vi "DataBuffer.vi"(0 "File Info In":T1={"FilePath"=path "/opticsmac/Users/Data", "Field (T)"=0.0, "Temperature (K)"=-1.0, "X-Axis"=enum."nm", "Center nm"=500.0, "Current Grating Density"=enum."600", "CCD Parameters"={"Exposure Time (s)"=0.2, "Offset"=0.0, "BkgrdCrct"=FALSE, "Shutter"=FALSE, "Mode"=enum."Regular", "Repetition"=4, "dt or s"=0.0}, "Operation Mode"=enum."NML Data Acquisition", "Exp Index"=0, "Index_repetition"=0, "Index"=0, "Current Detector"=enum."CCD-1024x256"} {"CCD Parameters"."dt or s" format="%#.6f"; "CCD Parameters"."Repetition" min=1; "CCD Parameters"."Offset" format="%#.2f"; "CCD Parameters"."Exposure Time (s)" min=0.02 max=6000.0 format="%#.2f"; "Center nm" format="%.2f"; "Temperature (K)" format="%.2f"; "Field (T)" format="%.2f"}, 1 "Plot Buffer Size":i32=10, 2 "Action":T7(ring) caption="Pass(0)/Write(1)/Read(2)/Init(3)", 3 "Read#":i32=1, 5 "Y Array In":dbl[](array[numeric])=[4.359859227115864, 4.389200892828675, 4.418863708420512, 4.448852482615925, 4.479172114380057, 4.509827594937488, 4.540824009842933, 4.572166541105726, 4.6038604693694944, 4.635911176148454, 4.668324146122441, 4.701104969491852, 4.734259344394734, 4.767793079387671, 4.801712095992179, 4.83602243130902, 4.870730240701915, 4.905841800553186, 4.941363511093324, 4.97730189930649, 5.0136636219147634, 5.050455468442887, 5.087684364366512, 5.125357374346244, 5.16348170554992, 5.202064711066347, 5.241113893412698, 5.280636908138933, 5.320641567532123, 5.361135844423454, 5.40212787610175, 5.443625968336108, 5.485638599511655, 5.528174424881744, 5.571242280940019, 5.614851189916724, 5.659010364402478, 5.703729212104152, 5.749017340736845, 5.79488456305601, 5.8413409020348865, 5.888396596191121, 5.936062105068024, 5.984348114875219, 6.033265544293544, 6.082825550450229, 6.133039535069095, 6.1839191508021365, 6.235476307748183, 6.287723180164464, 6.340672213378188, 6.394336130903802, 6.44872794177352, 6.5038609480878895, 6.55974875279337, 6.616405267695311, 6.673844721713221, 6.732081669387259, 6.79113099964405, 6.851007944830221, 6.9117280900235425, 6.9733073826300265, 7.0357621422775445, 7.099109071015688, 7.1633652638319365, 7.228548219495836, 7.294675851741292, 7.36176650079951, 7.429838945294219, 7.498912414511272, 7.569006601056504, 7.640141673914049, 7.7123382919199805, 7.785617617665268, 7.860001331842512, 7.935511648052952, 8.012171328088485, 8.090003697706326, 8.169032662913095, 8.249282726775652, 8.33077900677827, 8.413547252743905, 8.49761386534048, 8.58300591519227, 8.66975116261715, 8.757878078012872, 8.847415862913794, 8.93839447174277, 9.030844634282277, 9.124797878889435, 9.220286556482478, 9.317343865324164, 9.41600387663149, 9.516301561040184, 9.618272815953393, 9.721954493806981, 9.827384431281825, 9.934601479497585, 10.043645535221685, 10.154557573128157, 10.267379679144385, 10.382155084921548, 10.498928203469083, 10.617744665992642, 10.738651359976075, 10.861696468551548, 10.986929511199559, 11.114401385825383, 11.244164412257609, 11.376272377215363, 11.510780580794803, 11.647745884522498, 11.787226761028752, 11.929283345392315, 12.073977488209161, 12.22137281044176, 12.371534760102007, 12.524530670826199, 12.680429822398747, 12.83930350328164, 13.001225075210728, 13.166270039915263, 13.33451610802253, 13.506043270206384, 13.680933870638214, 13.859272682802093, 14.041146987729777, 14.226646654715656, 14.41586422456719, 14.608894995444231, 14.80583711134241, 15.00679165326711, 15.211862733147012, 15.421157590528683, 15.634786692088575, 15.852863833997525, 16.075506247159804, 16.302834705347756, 16.534973636240313, 16.77205123536335, 17.014199582923293, 17.261554763504943, 17.51425698859712, 17.77245072188844, 18.036284807256397, 18.3059125993568, 18.58149209668873, 18.863186076991337, 19.15116223479378, 19.445593320905605, 19.746657283603096, 20.054537411216362, 20.369422475784297, 20.691506877387, 21.02099078870748, 21.35808029931693, 21.702987559097092, 22.0559309201451, 22.417135076413132, 22.786831200239348, 23.165257074828247, 23.552657221611106, 23.949283021300772, 24.35539282730692, 24.771252070023422, 25.197133350337953, 25.63331652051566, 26.080088750418582, 26.537744576792313, 27.006585933108887, 27.486922157200187, 27.979069973614642, 28.48335344733274, 29.000103905129734, 29.52965982050742, 30.072366657732513, 30.628576670076946, 31.198648646914766, 31.78294760382926, 32.38184440935961, 32.99571534146977, 33.624941566211746, 34.26990853044752, 34.931005259824005, 35.60862355250491, 36.3031570584605, 37.01500023335454, 37.74454715533088, 38.49219019221989, 39.25831850591429, 40.04331637991872, 40.847561355318334, 41.67142215974196, 42.51525641324812, 43.37940809451772, 44.26420475032537, 45.169954430957425, 46.09694233418251, 47.04542714051036, 48.015637022906574, 49.00776531492666, 50.02196582239054, 51.05834776541544, 52.11697033983435, 53.19783688989854, 54.30088868779076, 55.42599831987955, 56.57296268504168, 57.74149561674433, 58.931220148080584, 60.1416604476788, 61.37223346434939, 62.622240329675115, 63.890857580390986, 65.17712827640742, 66.4799531056599, 67.79808158341963, 69.1301034712415, 70.47444055896403, 71.82933897185566, 73.19286218368788, 74.56288493456158, 75.93708826921247, 77.31295592634606, 78.68777232151824, 80.05862237420615, 81.42239343285824, 82.77577954893358, 84.11528834098996, 85.43725067181454, 86.73783333448564, 88.0130549062849, 89.25880488223545, 90.4708661424704, 91.64494074005955, 92.77667891917588, 93.86171118887495, 94.89568318741601, 95.87429297840674, 96.79333032630886, 97.64871740856572, 98.43655033863818, 99.15314080272404, 99.79505705677101, 100.35916349333694, 100.84265797303367, 101.24310612502882, 101.55847185679316, 101.78714337508754, 101.92795410705088, 101.98019801980197, 101.94363896561752, 101.81851382289437, 101.60552935527126, 101.30585286653462, 100.92109688110092, 100.4532982230126, 99.90489199503531, 99.27868106899476, 98.57780178535918, 97.80568662187997, 96.96602462681605, 96.06272042200558, 95.09985256623146, 94.08163203227065, 93.01236149485176, 91.89639605523514, 90.73810594515385, 89.54184166257876, 88.31190189802533, 87.05250451647399, 85.76776076963034, 84.461652828644, 83.13801465065819, 81.8005161249856, 80.4526503871352, 79.09772414177037, 77.73885079871027, 76.37894619898024, 75.02072668985214, 73.66670929786417, 72.31921374603169, 70.98036606460397, 69.65210355285129, 68.33618086133153, 67.03417697891065, 65.74750292571056, 64.47740997120414, 63.22499821536264, 61.99122538944135, 60.77691575122682, 59.582768967111335, 58.40936888981143, 57.25719215587677, 56.12661654114332, 55.017929024924804, 53.93133352507879, 52.86695827602707, 51.82486283053664, 50.80504467356964, 49.807445442875476, 48.831956756394504, 47.87842565094678, 46.94665964030745, 46.036431403641515, 45.14748311748012, 44.27953044611727, 43.43226620646358, 42.6053637241895, 41.79847989842212, 41.011257992390064, 40.243330167348105, 39.49431977680977, 38.763843437704175, 38.05151289452863, 37.356936691921696, 36.67972167041139, 36.01947429933415, 35.37580186017517, 34.74831349280977, 34.13662111634363, 33.540340235512275, 32.959090642839186, 32.39249702604861, 31.840189489538492, 31.301803998049735, 30.7769827500592, 30.265374487814174, 29.76663475037882, 29.28042607553899, 28.80641815591104, 28.344287954158954, 27.893719781782664, 27.454405345555568, 27.026043765322786, 26.608341566525006, 26.201012650514798, 25.803778245431467, 25.41636684014538, 25.03851410354023, 24.669962791171823, 24.31046264115136, 23.95977026090333, 23.61764900628636, 23.28386885441087, 22.95820627133951, 22.640444075739502, 22.330371299429107, 22.027783045661604, 21.73248034589445, 21.444270015698585, 21.16296451039404, 20.888381780917932, 20.620345130372943, 20.35868307164673, 20.10322918643533, 19.853821985965663, 19.61030477366188, 19.372525509968213, 19.140336679507016, 18.913595160715975, 18.692162098089153, 18.475902777115053, 18.26468650198858, 18.058386476154528, 17.856879685719345, 17.660046785759945, 17.467771989538537, 17.279942960625498, 17.09645070792191, 16.917189483561163, 16.742056683667286, 16.570952751935298, 16.403781085997196, 16.240447946532107, 16.080862369071976, 15.924936078455998, 15.772583405879114, 15.623721208481035, 15.478268791420303, 15.336147832373733, 15.197282308405232, 15.061598425142755, 14.929024548204785, 14.799491136817574, 14.672930679561734, 14.549277632191464, 14.428468357465825, 14.310441066935024, 14.195135764625045, 14.08249419256267, 13.972459778087526, 13.864977582895126, 13.759994253758327, 13.657457974875705, 13.557318421794335, 13.459526716859063, 13.364035386138228, 13.27079831777925, 13.179770721748449, 13.090909090909092, 13.004171163395661, 12.91951588624077, 12.836903380214224, 12.75629490583483, 12.677652830515154, 12.600940596803213, 12.526122691683634, 12.453164616903683, 12.38203286029049, 12.312694868025606, 12.24511901784625, 12.179274593141457, 12.115131757913815, 12.05266153257834, 11.99183577056985, 11.932627135733041, 11.87500908046845, 11.818955824609674, 11.76444233500797, 11.711444305800104, 11.65993813933795, 11.60990092775727, 11.561310435165108, 11.514145080425847, 11.468383920525726, 11.424006634497912, 11.380993507889265, 11.339325417751663, 11.298983818141277, 11.259950726108972, 11.222208708166901, 11.185740867215678, 11.150530829917827, 11.116562734503766, 11.083821218996304, 11.052291409841342, 11.021958910931758, 10.992809793012693, 10.964830583456795, 10.938008256397914, 10.912330223212965, 10.887784323341283, 10.864358815431716, 10.842042368808027, 10.820824055243078, 10.800693341033405, 10.781640079365355, 10.763654502964759, 10.746727217022421, 10.730849192387653, 10.716011759022894, 10.702206599712252, 10.689425744017434, 10.677661562474725, 10.666906761026693, 10.657154375683012, 10.648397767404552, 10.640630617205472, 10.633846921468175, 10.628040987466086, 10.623207429089685, 10.619341162771164, 10.616437403603506, 10.61449166164985, 10.613499738439238, 10.613457723645045, 10.614361991942566, 10.616209200042398, 10.61899628389644, 10.622720456073516, 10.627379203301786, 10.632970284175236, 10.639491727021781, 10.646941827930538, 10.65531914893617, 10.664622516358094, 10.674851019292753, 10.68600400825716, 10.698081093981964, 10.711082146352725, 10.725007293497864, 10.73985692102218, 10.755631671384794, 10.77233244342051, 10.789960392003877, 10.808516927855083, 10.828003717487244, 10.848422683294594, 10.869776003781105, 10.892066113929618, 10.91529570571105, 10.939467728734005, 10.96458539103486, 10.990652160008423, 11.01767176347996, 11.045648190918651, 11.074585694793534, 11.104488792072516, 11.135362265865236, 11.167211167211168, 11.20004081701363, 11.233856808121402, 11.268665007559191, 11.304471558908258, 11.341282884839375, 11.379105689799312, 11.41794696285327, 11.457813980685149, 11.498714310757618, 11.540655814634878, 11.583646651469962, 11.62769528165972, 11.672810470670129, 11.719001293034513, 11.766277136528466, 11.814647706523917, 11.864123030526423, 11.914713462898968, 11.966429689775758, 12.019282734170648, 12.073283961283387, 12.12844508400873, 12.184778168652574, 12.242295640859474, 12.301010291757152, 12.360935284322133, 12.42208415997257, 12.48447084539341, 12.548109659599271, 12.613015321241827, 12.679202956166797, 12.746688105227863, 12.815486732363786, 12.885615232945288, 12.957090442399794, 13.029929645120367, 13.104150583667508, 13.179771468271484, 13.256810986643078, 13.335288314102453, 13.415223124033782, 13.496635598676047, 13.579546440259186, 13.66397688249509, 13.749948702434974, 13.837484232702424, 13.926606374114439, 14.017338608701486, 14.109705013137976, 14.203730272596845, 14.299439695039455, 14.396859225955392, 14.4960154635654, 14.596935674501095, 14.699647809977643, 14.804180522472912, 14.910563182930376, 15.018825898501593, 15.128999530844538, 15.241115714996932, 15.355206878840859, 15.471306263179047, 15.589447942441705, 15.709666846043369, 15.831998780412336, 15.956480451712276, 16.08314948928004, 16.212044469802226, 16.343204942253628, 16.47667145362424, 16.612485575458262, 16.750689931233456, 16.89132822460762, 17.034445268559747, 17.180087015457268, 17.328300588077308, 17.479134311615432, 17.632637746713556, 17.78886172353971, 17.9478583769566, 18.109681182812103, 18.274384995391078, 18.442026086065923, 18.612662183184362, 18.786352513237837, 18.963157843349737, 19.143140525129375, 19.326364539935806, 19.51289554559672, 19.70280092463277, 19.896149834033558, 20.09301325663871, 20.29346405417522, 20.49757702200397, 20.705428945633606, 20.917098659055448, 21.13266710496104, 21.35221739690145, 21.57583488344913, 21.803607214428858, 22.03562440927946, 22.27197892761611, 22.51276574206055, 22.758082413407966, 23.008029168205347, 23.262708978810554, 23.522227646009927, 23.786693884269244, 24.056219409693583, 24.3309190307785, 24.610910742027375, 24.896315820519412, 25.187258925508026, 25.483868201129862, 25.786275382310958, 26.09461590394749, 26.409029013447665, 26.729657886715053, 27.05664974765271, 27.39015599127249, 27.73033231048255, 28.077338826633632, 28.431340223896083, 28.79250588753546, 29.161010046158022, 29.537031917981217, 29.920755861189793, 30.31237152842447, 30.71207402544193, 31.120064073983663, 31.536548178868856, 31.961738799326668, 32.395854524562374, 32.83912025353589, 33.291767378922756, 33.75403397519474, 34.22616499074848, 34.70841244397801, 35.20103562315853, 35.70430128998762, 36.21848388658109, 36.743865745697, 37.2807373039094, 37.82939731740552, 38.39015308003834, 38.96332064319138, 39.54922503696516, 40.14820049211286, 40.76059066207344, 41.386748844375965, 42.0270382005743, 42.681831973785435, 43.35151370277646, 44.03647743141852, 44.73712791219888, 45.453880802309456, 46.18716285068311, 46.937412074152704, 47.705077920707076, 48.49062141761412, 49.29451530191956, 50.11724413059322, 50.95930436729756, 51.821204442444625, 52.70346478289072, 53.60661780723075, 54.53120788228832, 55.47779123595873, 56.44693582110416, 57.43922112472759, 58.45523791609419, 59.495587926931485, 60.56088345621398, 61.651746891388925, 62.76881013723119, 63.91271394274945, 65.08410711582407, 66.28364561441893, 67.51199150234996, 68.76981175672066, 70.05777691316518, 71.37655953411455, 72.72683248428955, 74.1092669966185, 75.52453051079203, 76.97328426561938, 78.45618062540582, 79.97386011959668, 81.52694817404465, 83.11605151148629, 84.7417541980828, 86.4046133123965, 88.10515421280739, 89.84386537927608, 91.62119280559367, 93.43753391876069, 95.29323100317171, 97.1885641087292, 99.12374342407416, 101.0989010989011, 103.11408250278154, 105.16923691237619, 107.26420762426427, 109.39872149710654, 111.5723779346085, 113.78463732972462, 116.03480900108816, 118.32203866462099, 120.64529549690151, 123.0033588622068, 125.39480479205825, 127.81799232482636, 130.27104983316252, 132.75186148874656, 135.25805403686783, 137.78698407721993, 140.33572607186628, 142.90106132583995, 145.47946820982128, 148.0671139170434, 150.65984806694533, 153.2531984854103, 155.84236950429036, 158.4222431302903, 160.98738343390016, 163.53204450143193, 166.05018227635358, 168.53547058854588, 170.9813216309795, 173.38091109184288, 175.72720808570307, 178.01300995009646, 180.23098188419874, 182.37370130512846, 184.43370668665264, 186.40355052675318, 188.27585596792636, 190.0433764705767, 191.6990578197283, 193.23610163304818, 194.64802943849332, 195.92874630773915, 197.0726029712699, 198.0744553067754, 198.92972008756837, 199.6344259043045, 200.1852582325435, 200.5795977101961, 200.81555081101075, 200.89197224975223, 200.80847862709987, 200.5654530119324, 200.16404035900476, 199.60613386401218, 198.89435255837313, 198.0320106357045, 197.02307917433632, 195.87214106971265, 194.58434011263304, 193.16532524079693, 191.6211910503684, 189.95841568084745, 188.18379718160273, 186.30438943418605, 184.32743864427007, 182.2603213348983, 180.11048467305204, 177.885389849312, 175.5924591102524, 173.23902691969622, 170.83229560237197, 168.37929570520407, 165.88685120068226, 163.3615495556608, 160.8097165991903, 158.23739604580024, 155.6503334662017, 153.0539644459122, 150.45340663317825, 147.85345535000155, 145.25858242321343, 142.67293788490863, 140.10035419216482, 137.5443526233475, 135.0081515211617, 132.4946760699316, 130.0065693149577, 127.54620415450763, 125.11569605897792, 122.71691629626862, 120.35150546699153, 118.0208871769936, 115.72628169770708, 113.46871948655841, 111.24905445988026, 109.06797692949733, 106.92602613107003, 104.82360228761749, 102.76097816526601, 100.7383100902379, 98.7556484066402, 96.81294736358653, 94.91007442793571, 93.04681902541851, 91.22290071827247, 89.43797683196064, 87.69164954700636, 85.98347247475698, 84.31295673795266, 82.67957657842356, 81.08277451527354, 79.52196607740966, 77.99654413451097, 76.50588285043271, 75.04934128267388, 73.62626665105351, 72.23599729800955, 70.87786536216365, 69.55119918590644, 68.25532547678353, 66.989571241518, 65.75326551045683, 64.54574086924336, 63.36633481351214, 62.21439094139057, 61.089259997666595, 59.99030078251254, 58.91688093678181, 57.8683776150366, 56.84417805662603, 55.84368006439242, 54.86629239981791, 53.911435102754524, 52.97853974323218, 52.06704961221306, 51.17641985762386, 50.306117571439195, 49.45562183311679, 48.624423714227504, 47.812026248683935, 47.01794437260552, 46.24170483747118, 45.48284609989282, 44.74091819103539, 44.01548256841131, 43.306111952540896, 42.61239015070839, 41.933911869839505, 41.270282520325516, 40.62111801242236, 39.986044546706715, 39.364698399897456, 38.75672570722455, 38.16178224240005, 37.579533196118035, 37.0096529539243, 36.451824874181916, 35.90574106678451, 35.37110217318958, 34.847617148262465, 34.335003044374055, 33.83298479812016, 33.341295019989, 32.85967378725514, 32.38786844032609, 31.92563338274469, 31.472729885000874, 31.028925892285255, 30.59399583628902, 30.167720451121262, 29.749886593406902, 29.340287066594833, 28.938720449497826, 28.54499092906973, 28.15890813740441, 27.780286992941413, 27.408947545840558, 27.044714827486775, 26.687418704078205, 26.3368937342368, 25.992979030586355, 25.65551812522657, 25.324358839035185, 24.999353154726343, 24.680357093584345, 24.367230595799825, 24.059837404323954, 23.758044952161082, 23.461724253019675, 23.170749795234723, 22.884999438884304, 22.60435431601352, 22.328698733885684, 22.05792008118085, 21.791908737057103, 21.53055798299983, 21.27376391737627, 21.021425372619895, 20.773443834969687, 20.529723366686287, 20.290170530675923, 20.054694317446987, 19.82320607433054, 19.595619436897397, 19.371850262501688, 19.151816565889344, 18.93543845680471, 18.722638079534455, 18.513339554329608, 18.30746892064386, 18.104954082134622, 17.90572475336819, 17.709712408176312, 17.51685022961275, 17.327073061456208, 17.140317361213445, 16.956521154571956, 16.77562399125692, 16.597566902248243, 16.42229235831149, 16.249744229803607, 16.07986774770962, 15.912609465871899, 15.747917224374362, 15.585740114042, 15.4260284420226, 15.26873369841338, 15.113808523899822, 14.961206678374843, 14.810883010504563, 14.662793428212746, 14.51689487005212, 14.373145277435007, 14.231503567696258, 14.091929607959841, 13.954384189785666, 13.818829004569535, 13.685226619673003, 13.553540455260446, 13.423734761818881, 13.295774598341003, 13.169625811148363, 13.045255013335167, 12.922629564813562, 12.801717552939623, 12.682487773703725, 12.56490971346569, 12.448953531218253, 12.334590041362802, 12.221790696979657, 12.110527573579299, 12.000773353317886, 11.892501309663155, 11.785685292497277, 11.68029971364149, 11.5763195327913, 11.4737202438479, 11.372477861634222, 11.272568908984288, 11.173970404192929, 11.076659848816483, 10.980615215812294, 10.885814938007247, 10.792237896885748, 10.699863411686152, 10.608671228797805, 10.518641511448305, 10.429754829672692, 10.341992150556594, 10.255334828743806, 10.169764597201846, 10.085263558236575, 10.001814174748855, 9.919399261726573, 9.838001977963811, 9.757605818001839, 9.678194604284215, 9.599752479520156, 9.522263899250422, 9.445713624608777, 9.370086715274489, 9.295368522609328, 9.22154468297399, 9.148601111219307, 9.076523994345967, 9.00529978532927, 8.934915197103027, 8.865357196698499, 8.79661299953429, 8.728670063851933, 8.661516085294144, 8.595138991620736, 8.529526937558694, 8.464668299782959, 8.400551672023308, 8.337165860294927, 8.274499878248228, 8.212542942635004, 8.151284468887964, 8.090714066809685, 8.030821536368922, 7.971596863600483, 7.913030216606138, 7.855111941654126, 7.797832559373704, 7.741182761043143, 7.685153404967791, 7.629735512946082, 7.574920266821415, 7.520699005116799, 7.467063219750945, 7.4140045528328695, 7.361514793533171, 7.309585875030267, 7.258209871528803, 7.207378995349226, 7.157085594085887, 7.107322147832155, 7.058081266471045, 7.009355687028948, 6.961138271091613, 6.913422002280089, 6.866199983785316] format="%.4f", 9 "File Info Buffer Init":T1[](array[typedef]) {"CCD Parameters"."dt or s" format="%#.6f"; "CCD Parameters"."Repetition" min=1; "CCD Parameters"."Offset" format="%#.2f"; "CCD Parameters"."Exposure Time (s)" min=0.02 max=6000.0 format="%#.2f"; "Center nm" format="%.2f"; "Temperature (K)" format="%.2f"; "Field (T)" format="%.2f"}, 11 "Y Array Buffer Init":dbl[][](array[numeric])=array1024x100[102400 elements] format="%.2f") -> (4 "File Info Out":T1={"FilePath"=path "/DATA/Labview Items", "Field (T)"=55.0, "Temperature (K)"=77.0, "X-Axis"=enum."nm", "Center nm"=55.0, "Current Grating Density"=enum."600", "CCD Parameters"={"Exposure Time (s)"=0.2, "Offset"=0.0, "BkgrdCrct"=FALSE, "Shutter"=FALSE, "Mode"=enum."Regular", "Repetition"=4, "dt or s"=0.0}, "Operation Mode"=enum."NML Data Acquisition", "Exp Index"=0, "Index_repetition"=0, "Index"=0, "Current Detector"=enum."CCD-1024x256"} {"CCD Parameters"."dt or s" format="%#.6f"; "CCD Parameters"."Repetition" min=1; "CCD Parameters"."Offset" format="%#.2f"; "CCD Parameters"."Exposure Time (s)" min=0.02 max=6000.0 format="%#.2f"; "Center nm" format="%.2f"; "Temperature (K)" format="%.2f"; "Field (T)" format="%.2f"}, 6 "Y Array out":dbl[](array[numeric])=[4.359859227115864, 4.389200892828675, 4.418863708420512, 4.448852482615925, 4.479172114380057, 4.509827594937488, 4.540824009842933, 4.572166541105726, 4.6038604693694944, 4.635911176148454, 4.668324146122441, 4.701104969491852, 4.734259344394734, 4.767793079387671, 4.801712095992179, 4.83602243130902, 4.870730240701915, 4.905841800553186, 4.941363511093324, 4.97730189930649, 5.0136636219147634, 5.050455468442887, 5.087684364366512, 5.125357374346244, 5.16348170554992, 5.202064711066347, 5.241113893412698, 5.280636908138933, 5.320641567532123, 5.361135844423454, 5.40212787610175, 5.443625968336108, 5.485638599511655, 5.528174424881744, 5.571242280940019, 5.614851189916724, 5.659010364402478, 5.703729212104152, 5.749017340736845, 5.79488456305601, 5.8413409020348865, 5.888396596191121, 5.936062105068024, 5.984348114875219, 6.033265544293544, 6.082825550450229, 6.133039535069095, 6.1839191508021365, 6.235476307748183, 6.287723180164464, 6.340672213378188, 6.394336130903802, 6.44872794177352, 6.5038609480878895, 6.55974875279337, 6.616405267695311, 6.673844721713221, 6.732081669387259, 6.79113099964405, 6.851007944830221, 6.9117280900235425, 6.9733073826300265, 7.0357621422775445, 7.099109071015688, 7.1633652638319365, 7.228548219495836, 7.294675851741292, 7.36176650079951, 7.429838945294219, 7.498912414511272, 7.569006601056504, 7.640141673914049, 7.7123382919199805, 7.785617617665268, 7.860001331842512, 7.935511648052952, 8.012171328088485, 8.090003697706326, 8.169032662913095, 8.249282726775652, 8.33077900677827, 8.413547252743905, 8.49761386534048, 8.58300591519227, 8.66975116261715, 8.757878078012872, 8.847415862913794, 8.93839447174277, 9.030844634282277, 9.124797878889435, 9.220286556482478, 9.317343865324164, 9.41600387663149, 9.516301561040184, 9.618272815953393, 9.721954493806981, 9.827384431281825, 9.934601479497585, 10.043645535221685, 10.154557573128157, 10.267379679144385, 10.382155084921548, 10.498928203469083, 10.617744665992642, 10.738651359976075, 10.861696468551548, 10.986929511199559, 11.114401385825383, 11.244164412257609, 11.376272377215363, 11.510780580794803, 11.647745884522498, 11.787226761028752, 11.929283345392315, 12.073977488209161, 12.22137281044176, 12.371534760102007, 12.524530670826199, 12.680429822398747, 12.83930350328164, 13.001225075210728, 13.166270039915263, 13.33451610802253, 13.506043270206384, 13.680933870638214, 13.859272682802093, 14.041146987729777, 14.226646654715656, 14.41586422456719, 14.608894995444231, 14.80583711134241, 15.00679165326711, 15.211862733147012, 15.421157590528683, 15.634786692088575, 15.852863833997525, 16.075506247159804, 16.302834705347756, 16.534973636240313, 16.77205123536335, 17.014199582923293, 17.261554763504943, 17.51425698859712, 17.77245072188844, 18.036284807256397, 18.3059125993568, 18.58149209668873, 18.863186076991337, 19.15116223479378, 19.445593320905605, 19.746657283603096, 20.054537411216362, 20.369422475784297, 20.691506877387, 21.02099078870748, 21.35808029931693, 21.702987559097092, 22.0559309201451, 22.417135076413132, 22.786831200239348, 23.165257074828247, 23.552657221611106, 23.949283021300772, 24.35539282730692, 24.771252070023422, 25.197133350337953, 25.63331652051566, 26.080088750418582, 26.537744576792313, 27.006585933108887, 27.486922157200187, 27.979069973614642, 28.48335344733274, 29.000103905129734, 29.52965982050742, 30.072366657732513, 30.628576670076946, 31.198648646914766, 31.78294760382926, 32.38184440935961, 32.99571534146977, 33.624941566211746, 34.26990853044752, 34.931005259824005, 35.60862355250491, 36.3031570584605, 37.01500023335454, 37.74454715533088, 38.49219019221989, 39.25831850591429, 40.04331637991872, 40.847561355318334, 41.67142215974196, 42.51525641324812, 43.37940809451772, 44.26420475032537, 45.169954430957425, 46.09694233418251, 47.04542714051036, 48.015637022906574, 49.00776531492666, 50.02196582239054, 51.05834776541544, 52.11697033983435, 53.19783688989854, 54.30088868779076, 55.42599831987955, 56.57296268504168, 57.74149561674433, 58.931220148080584, 60.1416604476788, 61.37223346434939, 62.622240329675115, 63.890857580390986, 65.17712827640742, 66.4799531056599, 67.79808158341963, 69.1301034712415, 70.47444055896403, 71.82933897185566, 73.19286218368788, 74.56288493456158, 75.93708826921247, 77.31295592634606, 78.68777232151824, 80.05862237420615, 81.42239343285824, 82.77577954893358, 84.11528834098996, 85.43725067181454, 86.73783333448564, 88.0130549062849, 89.25880488223545, 90.4708661424704, 91.64494074005955, 92.77667891917588, 93.86171118887495, 94.89568318741601, 95.87429297840674, 96.79333032630886, 97.64871740856572, 98.43655033863818, 99.15314080272404, 99.79505705677101, 100.35916349333694, 100.84265797303367, 101.24310612502882, 101.55847185679316, 101.78714337508754, 101.92795410705088, 101.98019801980197, 101.94363896561752, 101.81851382289437, 101.60552935527126, 101.30585286653462, 100.92109688110092, 100.4532982230126, 99.90489199503531, 99.27868106899476, 98.57780178535918, 97.80568662187997, 96.96602462681605, 96.06272042200558, 95.09985256623146, 94.08163203227065, 93.01236149485176, 91.89639605523514, 90.73810594515385, 89.54184166257876, 88.31190189802533, 87.05250451647399, 85.76776076963034, 84.461652828644, 83.13801465065819, 81.8005161249856, 80.4526503871352, 79.09772414177037, 77.73885079871027, 76.37894619898024, 75.02072668985214, 73.66670929786417, 72.31921374603169, 70.98036606460397, 69.65210355285129, 68.33618086133153, 67.03417697891065, 65.74750292571056, 64.47740997120414, 63.22499821536264, 61.99122538944135, 60.77691575122682, 59.582768967111335, 58.40936888981143, 57.25719215587677, 56.12661654114332, 55.017929024924804, 53.93133352507879, 52.86695827602707, 51.82486283053664, 50.80504467356964, 49.807445442875476, 48.831956756394504, 47.87842565094678, 46.94665964030745, 46.036431403641515, 45.14748311748012, 44.27953044611727, 43.43226620646358, 42.6053637241895, 41.79847989842212, 41.011257992390064, 40.243330167348105, 39.49431977680977, 38.763843437704175, 38.05151289452863, 37.356936691921696, 36.67972167041139, 36.01947429933415, 35.37580186017517, 34.74831349280977, 34.13662111634363, 33.540340235512275, 32.959090642839186, 32.39249702604861, 31.840189489538492, 31.301803998049735, 30.7769827500592, 30.265374487814174, 29.76663475037882, 29.28042607553899, 28.80641815591104, 28.344287954158954, 27.893719781782664, 27.454405345555568, 27.026043765322786, 26.608341566525006, 26.201012650514798, 25.803778245431467, 25.41636684014538, 25.03851410354023, 24.669962791171823, 24.31046264115136, 23.95977026090333, 23.61764900628636, 23.28386885441087, 22.95820627133951, 22.640444075739502, 22.330371299429107, 22.027783045661604, 21.73248034589445, 21.444270015698585, 21.16296451039404, 20.888381780917932, 20.620345130372943, 20.35868307164673, 20.10322918643533, 19.853821985965663, 19.61030477366188, 19.372525509968213, 19.140336679507016, 18.913595160715975, 18.692162098089153, 18.475902777115053, 18.26468650198858, 18.058386476154528, 17.856879685719345, 17.660046785759945, 17.467771989538537, 17.279942960625498, 17.09645070792191, 16.917189483561163, 16.742056683667286, 16.570952751935298, 16.403781085997196, 16.240447946532107, 16.080862369071976, 15.924936078455998, 15.772583405879114, 15.623721208481035, 15.478268791420303, 15.336147832373733, 15.197282308405232, 15.061598425142755, 14.929024548204785, 14.799491136817574, 14.672930679561734, 14.549277632191464, 14.428468357465825, 14.310441066935024, 14.195135764625045, 14.08249419256267, 13.972459778087526, 13.864977582895126, 13.759994253758327, 13.657457974875705, 13.557318421794335, 13.459526716859063, 13.364035386138228, 13.27079831777925, 13.179770721748449, 13.090909090909092, 13.004171163395661, 12.91951588624077, 12.836903380214224, 12.75629490583483, 12.677652830515154, 12.600940596803213, 12.526122691683634, 12.453164616903683, 12.38203286029049, 12.312694868025606, 12.24511901784625, 12.179274593141457, 12.115131757913815, 12.05266153257834, 11.99183577056985, 11.932627135733041, 11.87500908046845, 11.818955824609674, 11.76444233500797, 11.711444305800104, 11.65993813933795, 11.60990092775727, 11.561310435165108, 11.514145080425847, 11.468383920525726, 11.424006634497912, 11.380993507889265, 11.339325417751663, 11.298983818141277, 11.259950726108972, 11.222208708166901, 11.185740867215678, 11.150530829917827, 11.116562734503766, 11.083821218996304, 11.052291409841342, 11.021958910931758, 10.992809793012693, 10.964830583456795, 10.938008256397914, 10.912330223212965, 10.887784323341283, 10.864358815431716, 10.842042368808027, 10.820824055243078, 10.800693341033405, 10.781640079365355, 10.763654502964759, 10.746727217022421, 10.730849192387653, 10.716011759022894, 10.702206599712252, 10.689425744017434, 10.677661562474725, 10.666906761026693, 10.657154375683012, 10.648397767404552, 10.640630617205472, 10.633846921468175, 10.628040987466086, 10.623207429089685, 10.619341162771164, 10.616437403603506, 10.61449166164985, 10.613499738439238, 10.613457723645045, 10.614361991942566, 10.616209200042398, 10.61899628389644, 10.622720456073516, 10.627379203301786, 10.632970284175236, 10.639491727021781, 10.646941827930538, 10.65531914893617, 10.664622516358094, 10.674851019292753, 10.68600400825716, 10.698081093981964, 10.711082146352725, 10.725007293497864, 10.73985692102218, 10.755631671384794, 10.77233244342051, 10.789960392003877, 10.808516927855083, 10.828003717487244, 10.848422683294594, 10.869776003781105, 10.892066113929618, 10.91529570571105, 10.939467728734005, 10.96458539103486, 10.990652160008423, 11.01767176347996, 11.045648190918651, 11.074585694793534, 11.104488792072516, 11.135362265865236, 11.167211167211168, 11.20004081701363, 11.233856808121402, 11.268665007559191, 11.304471558908258, 11.341282884839375, 11.379105689799312, 11.41794696285327, 11.457813980685149, 11.498714310757618, 11.540655814634878, 11.583646651469962, 11.62769528165972, 11.672810470670129, 11.719001293034513, 11.766277136528466, 11.814647706523917, 11.864123030526423, 11.914713462898968, 11.966429689775758, 12.019282734170648, 12.073283961283387, 12.12844508400873, 12.184778168652574, 12.242295640859474, 12.301010291757152, 12.360935284322133, 12.42208415997257, 12.48447084539341, 12.548109659599271, 12.613015321241827, 12.679202956166797, 12.746688105227863, 12.815486732363786, 12.885615232945288, 12.957090442399794, 13.029929645120367, 13.104150583667508, 13.179771468271484, 13.256810986643078, 13.335288314102453, 13.415223124033782, 13.496635598676047, 13.579546440259186, 13.66397688249509, 13.749948702434974, 13.837484232702424, 13.926606374114439, 14.017338608701486, 14.109705013137976, 14.203730272596845, 14.299439695039455, 14.396859225955392, 14.4960154635654, 14.596935674501095, 14.699647809977643, 14.804180522472912, 14.910563182930376, 15.018825898501593, 15.128999530844538, 15.241115714996932, 15.355206878840859, 15.471306263179047, 15.589447942441705, 15.709666846043369, 15.831998780412336, 15.956480451712276, 16.08314948928004, 16.212044469802226, 16.343204942253628, 16.47667145362424, 16.612485575458262, 16.750689931233456, 16.89132822460762, 17.034445268559747, 17.180087015457268, 17.328300588077308, 17.479134311615432, 17.632637746713556, 17.78886172353971, 17.9478583769566, 18.109681182812103, 18.274384995391078, 18.442026086065923, 18.612662183184362, 18.786352513237837, 18.963157843349737, 19.143140525129375, 19.326364539935806, 19.51289554559672, 19.70280092463277, 19.896149834033558, 20.09301325663871, 20.29346405417522, 20.49757702200397, 20.705428945633606, 20.917098659055448, 21.13266710496104, 21.35221739690145, 21.57583488344913, 21.803607214428858, 22.03562440927946, 22.27197892761611, 22.51276574206055, 22.758082413407966, 23.008029168205347, 23.262708978810554, 23.522227646009927, 23.786693884269244, 24.056219409693583, 24.3309190307785, 24.610910742027375, 24.896315820519412, 25.187258925508026, 25.483868201129862, 25.786275382310958, 26.09461590394749, 26.409029013447665, 26.729657886715053, 27.05664974765271, 27.39015599127249, 27.73033231048255, 28.077338826633632, 28.431340223896083, 28.79250588753546, 29.161010046158022, 29.537031917981217, 29.920755861189793, 30.31237152842447, 30.71207402544193, 31.120064073983663, 31.536548178868856, 31.961738799326668, 32.395854524562374, 32.83912025353589, 33.291767378922756, 33.75403397519474, 34.22616499074848, 34.70841244397801, 35.20103562315853, 35.70430128998762, 36.21848388658109, 36.743865745697, 37.2807373039094, 37.82939731740552, 38.39015308003834, 38.96332064319138, 39.54922503696516, 40.14820049211286, 40.76059066207344, 41.386748844375965, 42.0270382005743, 42.681831973785435, 43.35151370277646, 44.03647743141852, 44.73712791219888, 45.453880802309456, 46.18716285068311, 46.937412074152704, 47.705077920707076, 48.49062141761412, 49.29451530191956, 50.11724413059322, 50.95930436729756, 51.821204442444625, 52.70346478289072, 53.60661780723075, 54.53120788228832, 55.47779123595873, 56.44693582110416, 57.43922112472759, 58.45523791609419, 59.495587926931485, 60.56088345621398, 61.651746891388925, 62.76881013723119, 63.91271394274945, 65.08410711582407, 66.28364561441893, 67.51199150234996, 68.76981175672066, 70.05777691316518, 71.37655953411455, 72.72683248428955, 74.1092669966185, 75.52453051079203, 76.97328426561938, 78.45618062540582, 79.97386011959668, 81.52694817404465, 83.11605151148629, 84.7417541980828, 86.4046133123965, 88.10515421280739, 89.84386537927608, 91.62119280559367, 93.43753391876069, 95.29323100317171, 97.1885641087292, 99.12374342407416, 101.0989010989011, 103.11408250278154, 105.16923691237619, 107.26420762426427, 109.39872149710654, 111.5723779346085, 113.78463732972462, 116.03480900108816, 118.32203866462099, 120.64529549690151, 123.0033588622068, 125.39480479205825, 127.81799232482636, 130.27104983316252, 132.75186148874656, 135.25805403686783, 137.78698407721993, 140.33572607186628, 142.90106132583995, 145.47946820982128, 148.0671139170434, 150.65984806694533, 153.2531984854103, 155.84236950429036, 158.4222431302903, 160.98738343390016, 163.53204450143193, 166.05018227635358, 168.53547058854588, 170.9813216309795, 173.38091109184288, 175.72720808570307, 178.01300995009646, 180.23098188419874, 182.37370130512846, 184.43370668665264, 186.40355052675318, 188.27585596792636, 190.0433764705767, 191.6990578197283, 193.23610163304818, 194.64802943849332, 195.92874630773915, 197.0726029712699, 198.0744553067754, 198.92972008756837, 199.6344259043045, 200.1852582325435, 200.5795977101961, 200.81555081101075, 200.89197224975223, 200.80847862709987, 200.5654530119324, 200.16404035900476, 199.60613386401218, 198.89435255837313, 198.0320106357045, 197.02307917433632, 195.87214106971265, 194.58434011263304, 193.16532524079693, 191.6211910503684, 189.95841568084745, 188.18379718160273, 186.30438943418605, 184.32743864427007, 182.2603213348983, 180.11048467305204, 177.885389849312, 175.5924591102524, 173.23902691969622, 170.83229560237197, 168.37929570520407, 165.88685120068226, 163.3615495556608, 160.8097165991903, 158.23739604580024, 155.6503334662017, 153.0539644459122, 150.45340663317825, 147.85345535000155, 145.25858242321343, 142.67293788490863, 140.10035419216482, 137.5443526233475, 135.0081515211617, 132.4946760699316, 130.0065693149577, 127.54620415450763, 125.11569605897792, 122.71691629626862, 120.35150546699153, 118.0208871769936, 115.72628169770708, 113.46871948655841, 111.24905445988026, 109.06797692949733, 106.92602613107003, 104.82360228761749, 102.76097816526601, 100.7383100902379, 98.7556484066402, 96.81294736358653, 94.91007442793571, 93.04681902541851, 91.22290071827247, 89.43797683196064, 87.69164954700636, 85.98347247475698, 84.31295673795266, 82.67957657842356, 81.08277451527354, 79.52196607740966, 77.99654413451097, 76.50588285043271, 75.04934128267388, 73.62626665105351, 72.23599729800955, 70.87786536216365, 69.55119918590644, 68.25532547678353, 66.989571241518, 65.75326551045683, 64.54574086924336, 63.36633481351214, 62.21439094139057, 61.089259997666595, 59.99030078251254, 58.91688093678181, 57.8683776150366, 56.84417805662603, 55.84368006439242, 54.86629239981791, 53.911435102754524, 52.97853974323218, 52.06704961221306, 51.17641985762386, 50.306117571439195, 49.45562183311679, 48.624423714227504, 47.812026248683935, 47.01794437260552, 46.24170483747118, 45.48284609989282, 44.74091819103539, 44.01548256841131, 43.306111952540896, 42.61239015070839, 41.933911869839505, 41.270282520325516, 40.62111801242236, 39.986044546706715, 39.364698399897456, 38.75672570722455, 38.16178224240005, 37.579533196118035, 37.0096529539243, 36.451824874181916, 35.90574106678451, 35.37110217318958, 34.847617148262465, 34.335003044374055, 33.83298479812016, 33.341295019989, 32.85967378725514, 32.38786844032609, 31.92563338274469, 31.472729885000874, 31.028925892285255, 30.59399583628902, 30.167720451121262, 29.749886593406902, 29.340287066594833, 28.938720449497826, 28.54499092906973, 28.15890813740441, 27.780286992941413, 27.408947545840558, 27.044714827486775, 26.687418704078205, 26.3368937342368, 25.992979030586355, 25.65551812522657, 25.324358839035185, 24.999353154726343, 24.680357093584345, 24.367230595799825, 24.059837404323954, 23.758044952161082, 23.461724253019675, 23.170749795234723, 22.884999438884304, 22.60435431601352, 22.328698733885684, 22.05792008118085, 21.791908737057103, 21.53055798299983, 21.27376391737627, 21.021425372619895, 20.773443834969687, 20.529723366686287, 20.290170530675923, 20.054694317446987, 19.82320607433054, 19.595619436897397, 19.371850262501688, 19.151816565889344, 18.93543845680471, 18.722638079534455, 18.513339554329608, 18.30746892064386, 18.104954082134622, 17.90572475336819, 17.709712408176312, 17.51685022961275, 17.327073061456208, 17.140317361213445, 16.956521154571956, 16.77562399125692, 16.597566902248243, 16.42229235831149, 16.249744229803607, 16.07986774770962, 15.912609465871899, 15.747917224374362, 15.585740114042, 15.4260284420226, 15.26873369841338, 15.113808523899822, 14.961206678374843, 14.810883010504563, 14.662793428212746, 14.51689487005212, 14.373145277435007, 14.231503567696258, 14.091929607959841, 13.954384189785666, 13.818829004569535, 13.685226619673003, 13.553540455260446, 13.423734761818881, 13.295774598341003, 13.169625811148363, 13.045255013335167, 12.922629564813562, 12.801717552939623, 12.682487773703725, 12.56490971346569, 12.448953531218253, 12.334590041362802, 12.221790696979657, 12.110527573579299, 12.000773353317886, 11.892501309663155, 11.785685292497277, 11.68029971364149, 11.5763195327913, 11.4737202438479, 11.372477861634222, 11.272568908984288, 11.173970404192929, 11.076659848816483, 10.980615215812294, 10.885814938007247, 10.792237896885748, 10.699863411686152, 10.608671228797805, 10.518641511448305, 10.429754829672692, 10.341992150556594, 10.255334828743806, 10.169764597201846, 10.085263558236575, 10.001814174748855, 9.919399261726573, 9.838001977963811, 9.757605818001839, 9.678194604284215, 9.599752479520156, 9.522263899250422, 9.445713624608777, 9.370086715274489, 9.295368522609328, 9.22154468297399, 9.148601111219307, 9.076523994345967, 9.00529978532927, 8.934915197103027, 8.865357196698499, 8.79661299953429, 8.728670063851933, 8.661516085294144, 8.595138991620736, 8.529526937558694, 8.464668299782959, 8.400551672023308, 8.337165860294927, 8.274499878248228, 8.212542942635004, 8.151284468887964, 8.090714066809685, 8.030821536368922, 7.971596863600483, 7.913030216606138, 7.855111941654126, 7.797832559373704, 7.741182761043143, 7.685153404967791, 7.629735512946082, 7.574920266821415, 7.520699005116799, 7.467063219750945, 7.4140045528328695, 7.361514793533171, 7.309585875030267, 7.258209871528803, 7.207378995349226, 7.157085594085887, 7.107322147832155, 7.058081266471045, 7.009355687028948, 6.961138271091613, 6.913422002280089, 6.866199983785316] format="%.4f", 10 "File Info Buffer Out":T1[](array[typedef]) {"CCD Parameters"."dt or s" format="%#.6f"; "CCD Parameters"."Repetition" min=1; "CCD Parameters"."Offset" format="%#.2f"; "CCD Parameters"."Exposure Time (s)" min=0.02 max=6000.0 format="%#.2f"; "Center nm" format="%.2f"; "Temperature (K)" format="%.2f"; "Field (T)" format="%.2f"}, 14 "Current Buffer Size":i32=10, 15 "Y Array Buffer Out":dbl[][](array[numeric]) format="%.2f")   [LabVIEW 2024]
doc: "Write (FIFO) or retrieve (LIFO) data from the buffer.\n\nWhen write to the buffer, set the desired \"Buffer Size\" and run the VI several iterations. Notice that initially, the buffer grows to reach \"Buffer Size\" and then the input data flows from the last buffer element through to the zero element on each iteration (First In, First Out).\n\nWhen read from the buffer, set the Read# to the nth previous input data, i.e. counting reversely, with the most recent input counted as the 1st readout. If the input is out of current buffer size, an error is returned. (Last In, First Out)\n\n*******************\nY-Array Format: row-index changes y-data and column-index changes different set of y-data: i.e., 1024rows x eg 100 columns.s\n(1) Need to Initiate first before it can operate properly;\n(2) Write the experimental data in. Output the correct last 10 yData Array and FileInfoArray so we can process them later.\n(3) Read the indexed data and mix them with the latest 9 yData from the yDataArray INPUT. Note there is difference between \"write\" and \"read\". \"Write\" outputs the latest 10 yData measurements whereas \"read\" mixes its reading with an outside data input.\n(4) The passing mode can fetch the shift register locals so the entire data buffer can be read and output."
uses:
  Globals and TypeDefs/Type Definitions.llb/FileInfoParameter.ctt
  Globals and TypeDefs/Type Definitions.llb/Wavelength Unit.ctt
  Globals and TypeDefs/Type Definitions.llb/McPherson Grating Density.ctl
  Globals and TypeDefs/Type Definitions.llb/CCDParameter.ctt
  Globals and TypeDefs/Type Definitions.llb/OperationMode.ctt
  Globals and TypeDefs/Type Definitions.llb/ListOfDetectors.ctt
  Globals and TypeDefs/gGeneral.vi
panel:
  out "Y Array Buffer Out size(s)":i32[](array[numeric])
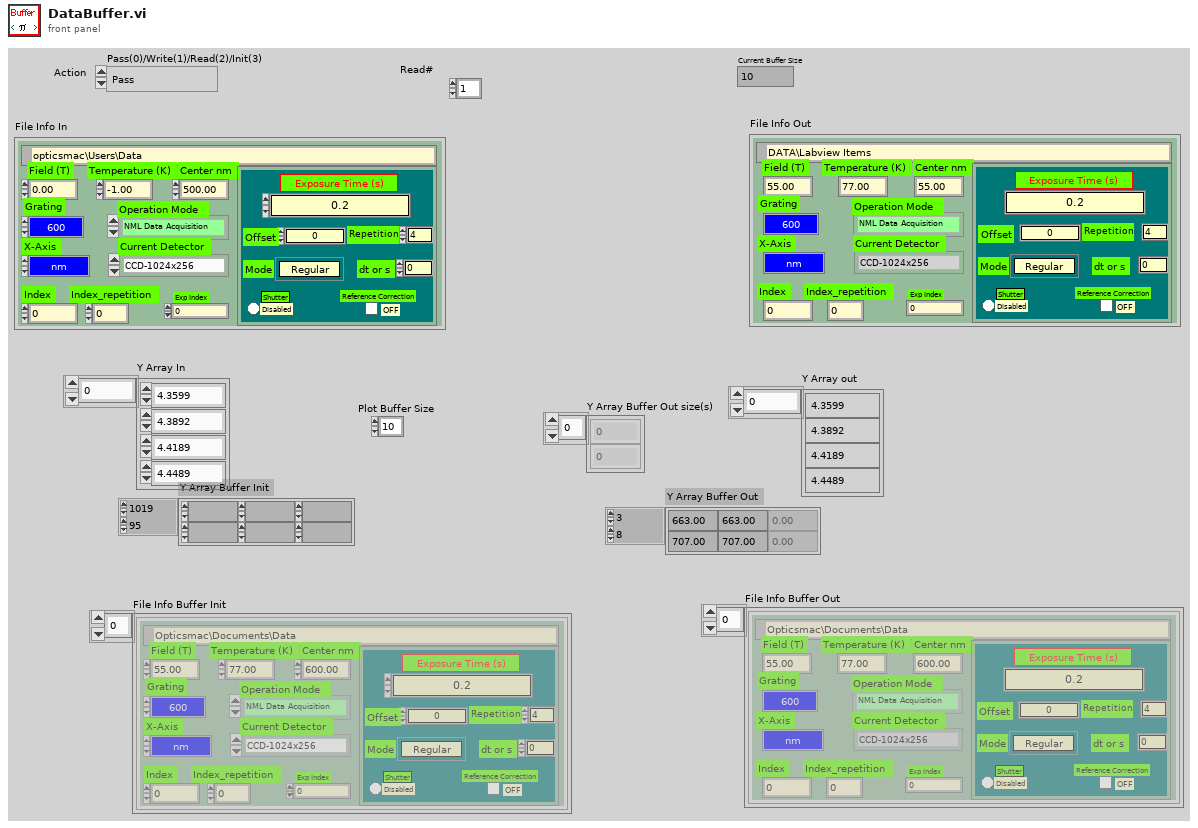
[diagram p1: front panel]
types:
  T1 = typedef "FileInfoParameter.ctt" = cluster{"FilePath":path, "Field (T)":dbl, "Temperature (K)":dbl, "X-Axis":T2, "Center nm":dbl, "Current Grating Density":T3, "CCD Parameters":T4, "Operation Mode":T5, "Exp Index":u32, "Index_repetition":u16, "Index":u16, "Current Detector":T6}
  T2 = typedef "Wavelength Unit.ctt" = enum8{"Point", "nm", "eV", "meV", "cm_1"}
  T3 = typedef "McPherson Grating Density.ctl" = enum8{"150", "300", "600", "1200", "1800"}
  T4 = typedef "CCDParameter.ctt" = cluster{"Exposure Time (s)":dbl, "Offset":dbl, "BkgrdCrct":bool, "Shutter":bool, "Mode":enum8{"Regular", "OverExp Cor", "SpikeRemove", "ForCalibration"}, "Repetition":u16, "dt or s":dbl}
  T5 = typedef "OperationMode.ctt" = enum16{"Standby", "CCD Single Shot", "CCD Sequence Shots", "CCD Custom Shots", "CCD Reference Shot", "Step Scanning ", "Time Scanning", "NML Data Acquisition"}
  T6 = typedef "ListOfDetectors.ctt" = enum8{"CCD-1024x256", "InGaAs PDA-1024x1", "CCD-1340x400", "Ge Single Channel", "Si Single Channel", "PMT Single Channel"}
  T7 = enum16{"Pass", "Write", "Read", "ReadPlotBlock", "Initialize", "InitFromBufferInput", "Resize Buffer"}
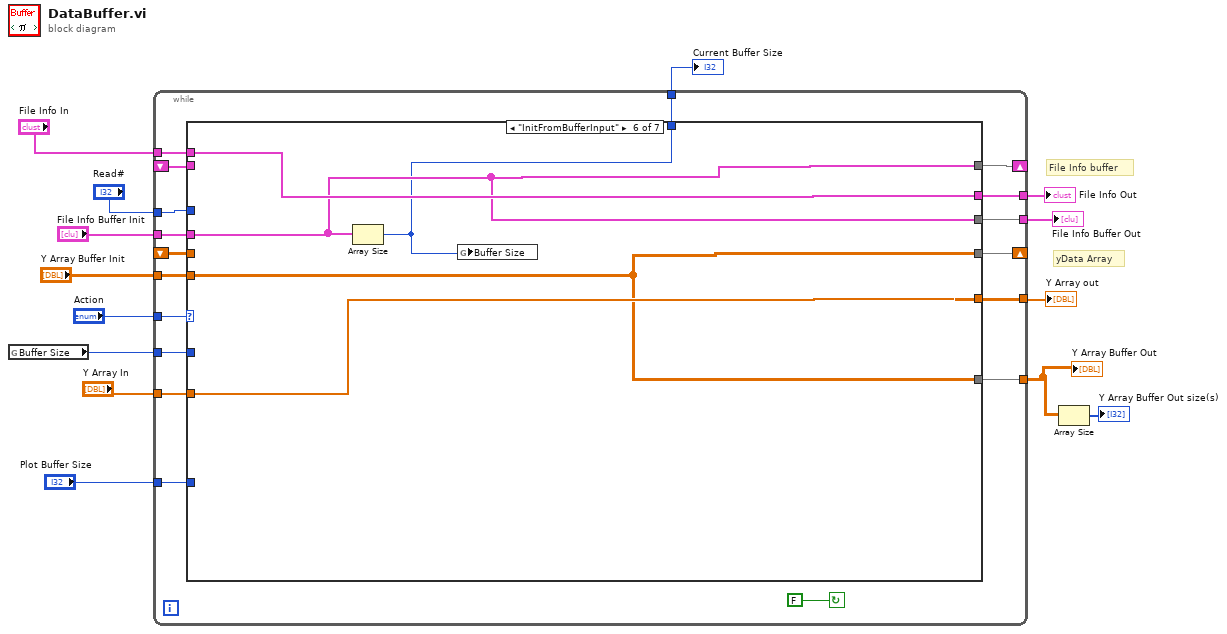
[diagram p0: block diagram]
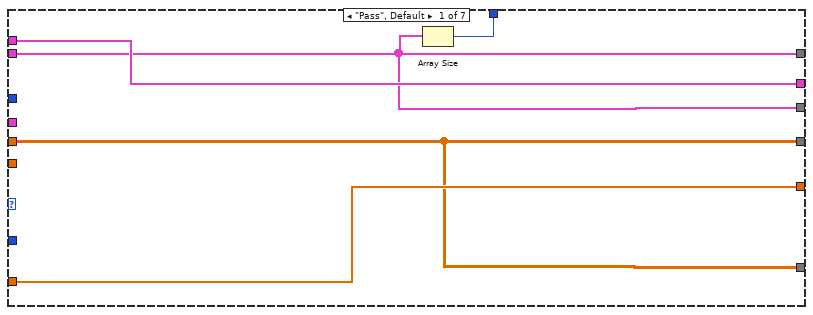
[diagram p2: hidden frame]
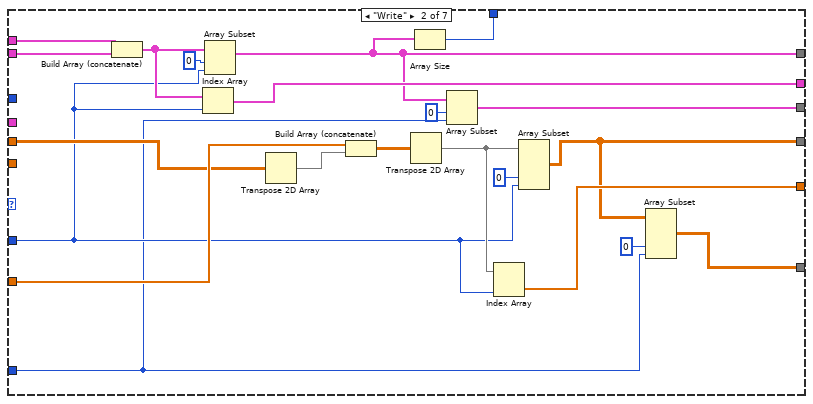
[diagram p3: hidden frame]
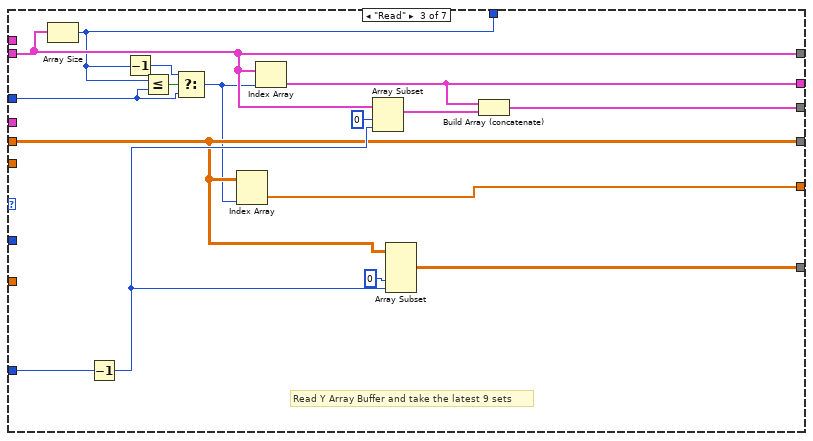
[diagram p4: hidden frame]
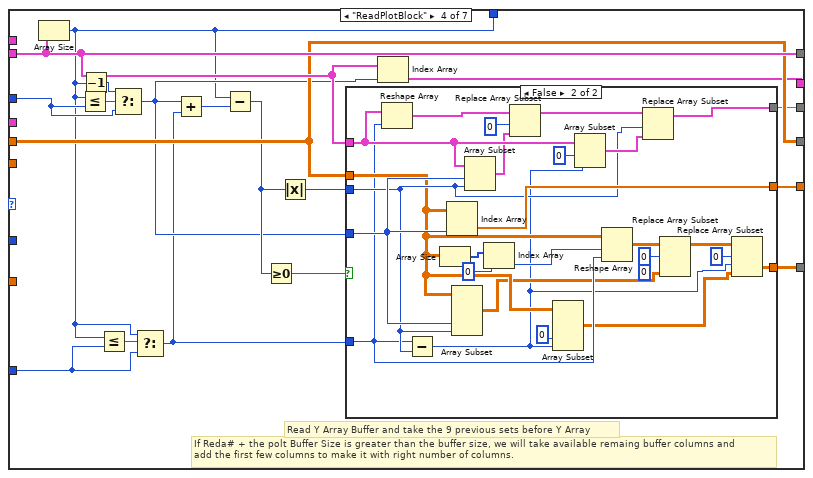
[diagram p5: hidden frame]
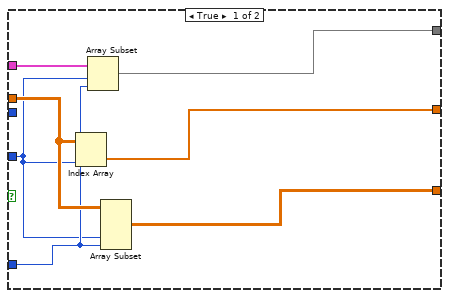
[diagram p6: hidden frame]
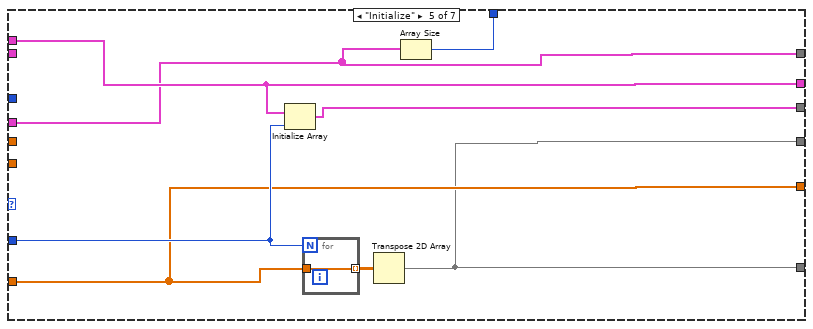
[diagram p7: hidden frame]
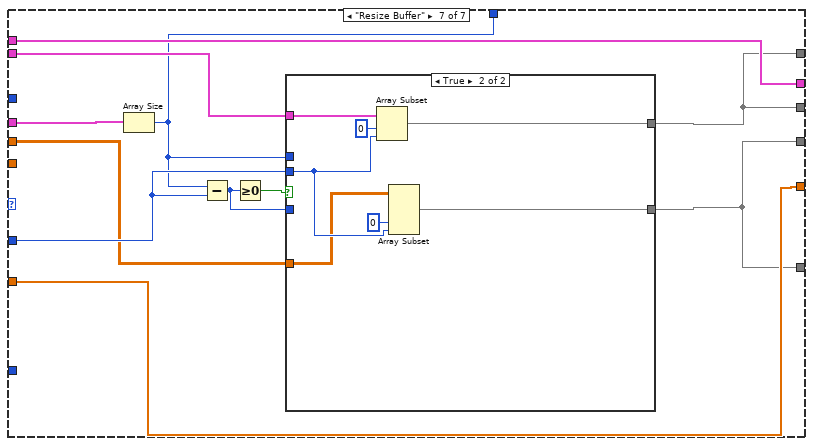
[diagram p8: hidden frame]
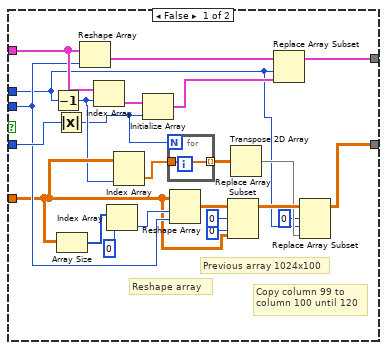
[diagram p9: hidden frame]
diagram:
  # "yData Array"
  # "File Info buffer"
  n1 = global read "gGeneral.vi" "Buffer Size"() -> (w3:u8)
  n2 = while {
    tunnel: "Read#" -> [w28]
    tunnel: [w32] -> w14
    tunnel: "File Info In" -> [w31]
    tunnel: "Action" -> [w30]
    shift-right: [w27] -> _
    shift-left: _ -> [w26]
    tunnel: [w25] -> w11
    tunnel: [w24] -> w10
    tunnel: "Y Array In" -> [w23]
    tunnel: [w22] -> w7
    tunnel: "Plot Buffer Size" -> [w21]
    tunnel: "Y Array Buffer Init" -> [w20]
    tunnel: w3 -> [w19]
    shift-right: [w18] -> _
    shift-left: _ -> [w16]
    tunnel: "File Info Buffer Init" -> [w17]
    tunnel: [w15] -> w1
    stop <- FALSE continue-if-true
    n3 = case shown="\"InitFromBufferInput\"" w30 {
      tunnel: w28 -> [_ _ w62 w81 _ _ _]
      tunnel: [w37 w58 w60 w76 w133 w135 w140] -> w32
      tunnel: w31 -> [w36 w56 _ _ w132 w137 w145]
      tunnel: [w34 w40 w65 w90 w126 w138 w143] -> w27
      tunnel: w26 -> [w34 w48 w65 w90 _ _ w147]
      tunnel: w16 -> [w33 w57 w69 w92 _ _ w149]
      tunnel: [w33 w52 w69 w92 w131 w136 w144] -> w18
      tunnel: [w36 w53 w72 w88 w132 w137 w145] -> w25
      tunnel: [w35 w42 w68 w91 w128 w139 w146] -> w24
      tunnel: w23 -> [w35 w49 _ _ w128 w139 w146]
      tunnel: [w33 w50 w71 w87 w130 w136 w144] -> w15
      tunnel: [w34 w38 w64 w89 w126 w138 w143] -> w22
      tunnel: w21 -> [_ w39 w70 w77 _ _ _]
      tunnel: w17 -> [_ _ _ _ w131 w136 w150]
      tunnel: w20 -> [_ _ _ _ _ w138 _]
      tunnel: w19 -> [_ w43 _ _ w129 _ w148]
      frame "Pass", Default {
        n4 = Array Size(array=w33) -> (size(s)=w37:i32)
      }
      frame "Write" {
        n5 = Build Array (concatenate)(w56, w57) -> (w54:T1[])
        n6 = Index Array(array=w54, index=w43) -> (element=w53:T1)
        n7 = Array Subset(array=w54, index=0, length=w43) -> (w52:T1[])
        n8 = Transpose 2D Array(2D array=w48) -> (transposed array=w47:dbl[][])
        n9 = Build Array (concatenate)(w49, w47) -> (w45:dbl[][])
        n10 = Transpose 2D Array(2D array=w45) -> (transposed array=w44:dbl[][])
        n11 = Array Size(array=w52) -> (size(s)=w58:i32)
        n12 = Array Subset(array=w52, index=0, length=w39) -> (w50:T1[])
        n13 = Index Array(array=w44, index (col)=w43) -> (element=w42:dbl[])  [unwired: 1 in]
        n14 = Array Subset(array=w44, index (col)=0 ("index"), length (col)=w43) -> (w40:dbl[][])  [unwired: 2 in]
        n15 = Array Subset(array=w40, index (col)=0 ("index"), length (col)=w39) -> (w38:dbl[][])  [unwired: 2 in]
      }
      frame "Read" {
        # "Read Y Array Buffer and take the latest 9 sets"
        n16 = Array Size(array=w69) -> (size(s)=w60:i32)
        n17 = Decrement(x=w70) -> (x-1=w67:i32)
        n18 = Decrement(x=w60) -> (x-1=w59:i32)
        n19 = Less Or Equal?(x=w60, y=w62) -> (x <= y?=w63:bool)
        n20 = Select(t=w59, s=w63, f=w62) -> (s? t:f=w61:i32)
        n21 = Index Array(array=w65, index (col)=w61) -> (element=w68:dbl[])  [unwired: 1 in]
        n22 = Index Array(array=w69, index=w61) -> (element=w72:T1)
        n23 = Array Subset(array=w69, index=0, length=w67) -> (w73:T1[])
        n24 = Array Subset(array=w65, index (col)=0 ("index"), length (col)=w67) -> (w64:dbl[][])  [unwired: 2 in]
        n25 = Build Array (concatenate)(w72, w73) -> (w71:T1[])
      }
      frame "ReadPlotBlock" {
        # "Read Y Array Buffer and take the 9 previous sets before Y Array"
        # "If Reda# + the polt Buffer Size is greater than the buffer size, we will take available remaing buffer columns and\nadd the first few columns to make it with right number of columns."
        n26 = Array Size(array=w92) -> (size(s)=w76:i32)
        n27 = Less Or Equal?(x=w76, y=w81) -> (x <= y?=w82:bool)
        n28 = Decrement(x=w76) -> (x-1=w79:i32)
        n29 = Less Or Equal?(x=w76, y=w77) -> (x <= y?=w78:bool)
        n30 = Select(t=w79, s=w82, f=w81) -> (s? t:f=w80:i32)
        n31 = Select(t=w76, s=w78, f=w77) -> (s? t:f=w75:i32)
        n32 = Add(x=w80, y=w75) -> (x+y=w86:i32)
        n33 = Subtract(x=w76, y=w86) -> (x-y=w84:i32)
        n34 = Greater Or Equal To 0?(x=w84) -> (x >= 0?=w85:bool)
        n35 = Absolute Value(x=w84) -> (abs(x)=w83:i32)
        n36 = case shown="False" w85 {
          tunnel: w92 -> [w99 w121]
          tunnel: [w98 w125] -> w91
          tunnel: w90 -> [w97 w111]
          tunnel: [w96 w102] -> w89
          tunnel: [w95 w114] -> w87
          tunnel: w80 -> [w93 w124]
          tunnel: w75 -> [w94 w109]
          tunnel: w83 -> [_ w115]
          frame True {
            n37 = Index Array(array=w97, index (col)=w93) -> (element=w98:dbl[])  [unwired: 1 in]
            n38 = Array Subset(array=w99, index=w93, length=w94) -> (w95:T1[])
            n39 = Array Subset(array=w97, index (col)=w93, length (col)=w94) -> (w96:dbl[][])  [unwired: 2 in]
          }
          frame False {
            n40 = Reshape Array(w121, w109) -> (w120:T1[])
            n41 = Subtract(x=w109, y=w115) -> (x-y=w100:i32)
            n42 = Array Size(array=w111) -> (size(s)=w113:i32[])
            n43 = Index Array(array=w111, index (col)=w124) -> (element=w125:dbl[])  [unwired: 1 in]
            n44 = Array Subset(array=w111, index (col)=w124, length (col)=w115) -> (w107:dbl[][])  [unwired: 2 in]
            n45 = Array Subset(array=w121, index=w124, length=w115) -> (w118:T1[])
            n46 = Index Array(array=w113, index=0) -> (element=w110:i32)
            n47 = Replace Array Subset(array=w120, new element=w118, index=0) -> (w117:T1[])
            n48 = Array Subset(array=w111, index (col)=0 ("index"), length (col)=w100) -> (w101:dbl[][])  [unwired: 2 in]
            n49 = Array Subset(array=w121, index=0, length=w100) -> (w116:T1[])
            n50 = Reshape Array(w111, w110, w109) -> (w108:dbl[][])
            n51 = Replace Array Subset(array=w117, new element=w116, index=w115) -> (w114:T1[])
            n52 = Replace Array Subset(array=w108, new element=w107, index (row)=0, index (col)=0 ("disabled index (col)")) -> (w103:dbl[][])
            n53 = Replace Array Subset(array=w103, new element=w101, index (row)=0, index (col)=w100) -> (w102:dbl[][])
          }
        }
        n54 = Index Array(array=w92, index=w80) -> (element=w88:T1)
      }
      frame "Initialize" {
        n55 = Initialize Array(w132, w129) -> (w130:T1[])
        n56 = for {
          N: w129 -> [_]
          tunnel: w128 -> [w134]
          tunnel: [w134] -> w127 mode=indexing
        }
        n57 = Transpose 2D Array(2D array=w127) -> (transposed array=w126:dbl[][])
        n58 = Array Size(array=w131) -> (size(s)=w133:i32)
      }
      frame "InitFromBufferInput" {
        n59 = Array Size(array=w136) -> (size(s)=w135:i32)
        n60 = global write "gGeneral.vi" "Buffer Size"(w135) -> ()
      }
      frame "Resize Buffer" {
        n61 = Array Size(array=w150) -> (size(s)=w140:i32)
        n62 = Subtract(x=w140, y=w148) -> (x-y=w141:i32)
        n63 = Greater Or Equal To 0?(x=w141) -> (x >= 0?=w142:bool)
        n64 = case shown="True" w142 {
          tunnel: w149 -> [w173 w181]
          tunnel: w148 -> [w164 w180]
          tunnel: w147 -> [w160 w179]
          tunnel: [w168 w176] -> w144
          tunnel: [w151 w175] -> w143
          tunnel: w140 -> [w152 _]
          tunnel: w141 -> [w171 _]
          frame False {
            # "Copy column 99 to\ncolumn 100 until 120"
            # "Previous array 1024x100"
            # "Reshape array"
            n65 = Decrement(x=w152) -> (x-1=w159:i32)
            n66 = Absolute Value(x=w171) -> (abs(x)=w158:i32)
            n67 = Array Size(array=w160) -> (size(s)=w167:i32[])
            n68 = Reshape Array(w173, w164) -> (w170:T1[])
            n69 = Index Array(array=w173, index=w159) -> (element=w172:T1)
            n70 = Index Array(array=w167, index=0) -> (element=w165:i32)
            n71 = Index Array(array=w160, index (col)=w159) -> (element=w157:dbl[])  [unwired: 1 in]
            n72 = Initialize Array(w172, w158) -> (w169:T1[])
            n73 = for {
              N: w158 -> [_]
              tunnel: w157 -> [w174]
              tunnel: [w174] -> w156 mode=indexing
            }
            n74 = Reshape Array(w160, w165, w164) -> (w163:dbl[][])
            n75 = Replace Array Subset(array=w163, new element=w160, index (row)=0, index (col)=0 ("disabled index (col)")) -> (w155:dbl[][])
            n76 = Transpose 2D Array(2D array=w156) -> (transposed array=w154:dbl[][])
            n77 = Replace Array Subset(array=w170, new element=w169, index=w152) -> (w168:T1[])
            n78 = Replace Array Subset(array=w155, new element=w154, index (row)=0, index (col)=w152) -> (w151:dbl[][])
          }
          frame True {
            n79 = Array Subset(array=w181, index=0, length=w180) -> (w176:T1[])
            n80 = Array Subset(array=w179, index (col)=0 ("index"), length (col)=w180) -> (w175:dbl[][])  [unwired: 2 in]
          }
        }
      }
    }
  }
  "Current Buffer Size" <- w14
  "Y Array Buffer Out" <- w7
  "File Info Buffer Out" <- w1
  "File Info Out" <- w11
  "Y Array out" <- w10
  n81 = Array Size(array=w7) -> (size(s)=→"Y Array Buffer Out size(s)":i32[])
